vi "Orion PDU Test Program Status.vi"(8 "error in (no error)":errorcluster) -> (0 "error out":errorcluster)   [LabVIEW 2024]
uses:
  <vilib>/httpClient/POSTBuffer.vi
  <vilib>/regexp/Match Regular Expression.xnode
  <vilib>/httpClient/LabVIEWHTTPClient.lvlib
panel:
  out "current":dbl
  out "x > 0?":bool[](array[boolean])
  out "array":dbl[](array[numeric])
  out "submatch 1":string
  out "body":string="<response>\r\n<pot0>,,6.1,0.0,0.0,0.0,0.0,0.0,0.0,0.0,0,1,1,1,0,0,0,0,1,0,0,0,0,0,0,0,1,0,0,0,0,0,0,0,0,5,5,5,5,5,5,5,6.1,0,</pot0>\r\n<outn>,,,,,,,,</outn>\r\n</response>\r\n"
  out "headers":string
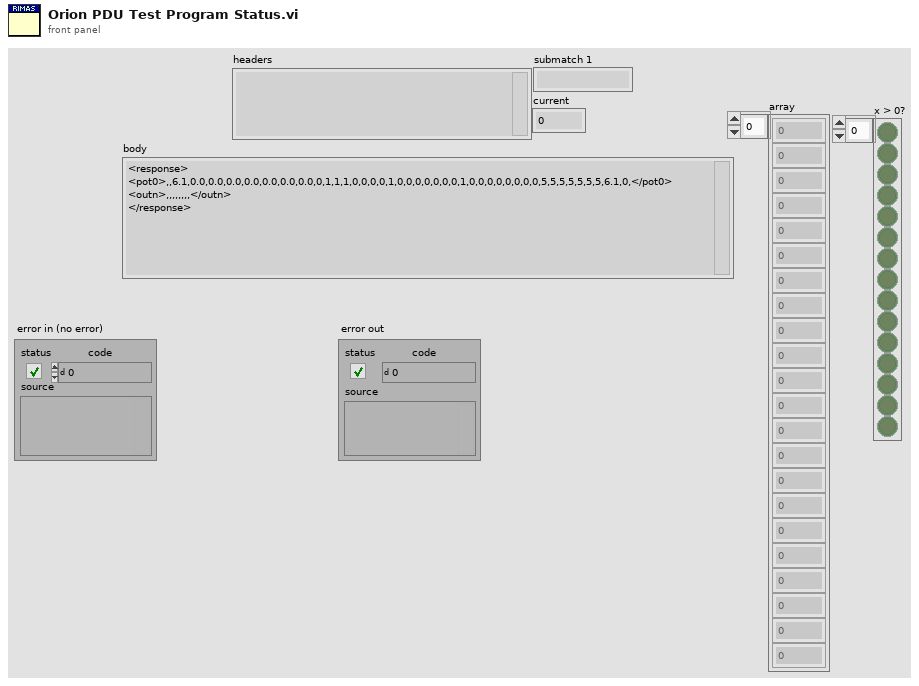
[diagram p1: front panel]
types:
  T1 = typedef "LabVIEWHTTPClient.lvlib/ClientHandle.ctl" = refnum<k1>
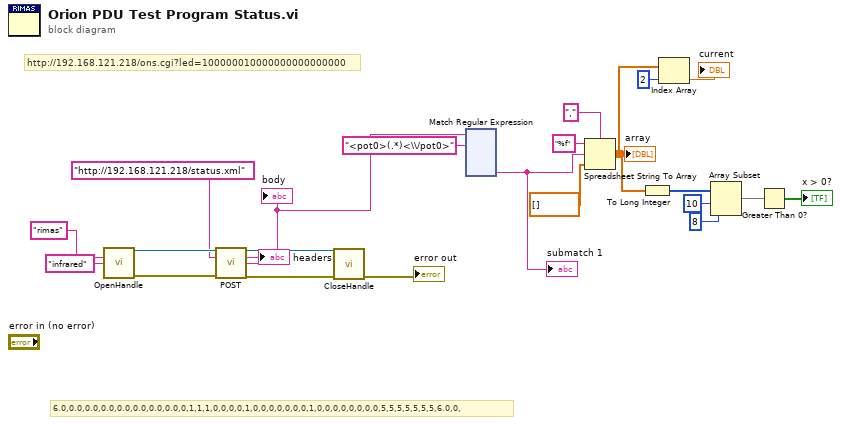
[diagram p0: block diagram]
diagram:
  # "6.0,0.0,0.0,0.0,0.0,0.0,0.0,0.0,0,1,1,1,0,0,0,0,1,0,0,0,0,0,0,0,1,0,0,0,0,0,0,0,0,5,5,5,5,5,5,5,6.0,0,"
  # "http://192.168.121.218/ons.cgi?led=100000010000000000000000"
  n1 = call <vilib>:"OpenHandle.vi"("username"="rimas", "password"="infrared") -> ("client handle out"=w23:T1, "error out"=w19:errorcluster)  [unwired: 12 in]
  n2 = call-poly <vilib>:"POST.vi"("client handle"=w23, "url"="http://192.168.121.218/status.xml", "error in (no error)"=w19) -> ("client handle out"=w21:T1, "headers"=→"headers":string, "body"=w14:string, "error out"=w20:errorcluster)  [unwired: 9 in]
  "body" <- w14
  n3 = call <vilib>:"CloseHandle.vi"("client handle"=w21, "error in (no error)"=w20) -> ("error out"=→"error out":errorcluster)  [unwired: 13 in]
  n4 = xnode "Match Regular Expression"("input string"=w14, "regular expression"="<pot0>(.*)<\\/pot0>") -> ("submatch 1"=w12:string)  [unwired: 4 in, 5 out]
  "submatch 1" <- w12
  n5 = Spreadsheet String To Array(delimiter (Tab)=",", format string="%f", spreadsheet string=w12, array type (2D Dbl)=dbl[] []) -> (array=w3:dbl[])
  "array" <- w3
  n6 = To Long Integer(number=w3) -> (32bit integer=w8:i32[])
  n7 = Index Array(array=w3, index=2) -> (element=→"current":dbl)
  n8 = Array Subset(array=w8, index=10, length=8) -> (w5:i32[])
  n9 = Greater Than 0?(x=w5) -> (x > 0?=→"x > 0?":bool[])
